vi "Machine Setting - ADC Parse Read Data (SubVI).vi"(11 "ADC":T1={"Active Ch"=[255, 255, 255, 0, 0, 0, 0, 0], "Filter Type"=2, "Post Filter"=[1, 1, 1, 1, 0, 200, 66, 184], "Gain"=[0, 0, 0, 0, 0, 122, 68, 0], "FS"=32, "IntOC"=0, "IntFC"=255, "SysOC"=255, "Cofficient"=[1.0, 1.0, 1.0, 1.0, 1.0, 1.0, 1.0, 1.0], "K"=[1.2450000047683716, 1.2450000047683716], "Max"=1048576}) -> (3 "Array":string[](array[string]))   [LabVIEW 2019]
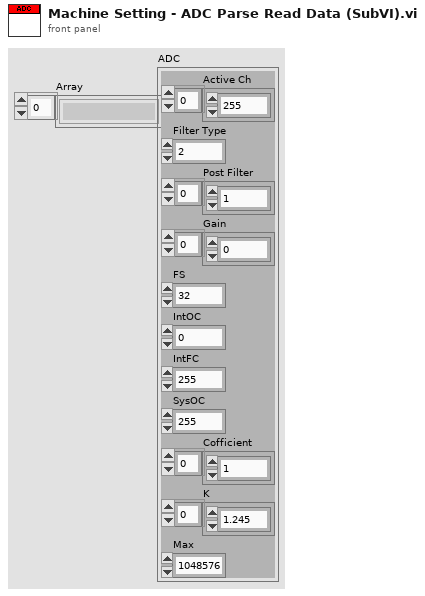
[diagram p1: front panel]
types:
  T1 = cluster{"Active Ch":u8[], "Filter Type":u8, "Post Filter":u8[], "Gain":u8[], "FS":u16, "IntOC":u8, "IntFC":u8, "SysOC":u8, "Cofficient":dbl[], "K":dbl[], "Max":i32}
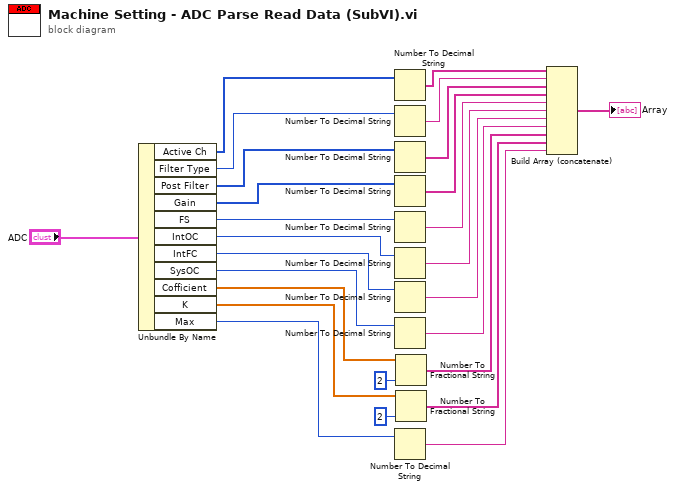
[diagram p0: block diagram]
diagram:
  n1 = Unbundle By Name("ADC") -> ("Active Ch"=w16:u8[], "Filter Type"=w15:u8, "Post Filter"=w14:u8[], "Gain"=w13:u8[], "FS"=w12:u16, "IntOC"=w11:u8, "IntFC"=w10:u8, "SysOC"=w9:u8, "Cofficient"=w8:dbl[], "K"=w7:dbl[], "Max"=w5:i32)
  n2 = Number To Decimal String(number=w16) -> (decimal integer string=w23:string[])  [unwired: 1 in]
  n3 = Number To Decimal String(number=w15) -> (decimal integer string=w22:string)  [unwired: 1 in]
  n4 = Number To Decimal String(number=w14) -> (decimal integer string=w21:string[])  [unwired: 1 in]
  n5 = Number To Decimal String(number=w13) -> (decimal integer string=w20:string[])  [unwired: 1 in]
  n6 = Number To Decimal String(number=w12) -> (decimal integer string=w19:string)  [unwired: 1 in]
  n7 = Number To Decimal String(number=w11) -> (decimal integer string=w18:string)  [unwired: 1 in]
  n8 = Number To Decimal String(number=w10) -> (decimal integer string=w17:string)  [unwired: 1 in]
  n9 = Number To Decimal String(number=w9) -> (decimal integer string=w4:string)  [unwired: 1 in]
  n10 = Number To Decimal String(number=w5) -> (decimal integer string=w1:string)  [unwired: 1 in]
  n11 = Number To Fractional String(number=w8, precision (6)=i16 2) -> (F-format string=w3:string[])  [unwired: 2 in]
  n12 = Number To Fractional String(number=w7, precision (6)=i16 2) -> (F-format string=w2:string[])  [unwired: 2 in]
  n13 = Build Array (concatenate)(w23, w22, w21, w20, w19, w18, w17, w4, w3, w2, w1) -> (→"Array":string[])
